vi "Analyze Condition C.vi"(6 "Conditions":T8, 8 "error in":errorcluster, 10 "PLC Data In":T1 {"PLC Data - LDO"."Timing"."Absolute Time" format="%<%H:%M:%S%3u>t"; "PLC Data - LDO"."Timing"."Display Time" format="%#.20f"; "PLC Data - LDO"."Timing"."Test Time Ref" format="%#.20f"; "PLC Data - LDO"."Timing"."Precondition Time Ref" format="%#.20f"; "PLC Data - LDO"."Timing"."First Call Time Ref" format="%#.20f"; "PLC Data - FVIR"."Timing"."Absolute Time" format="%<%H:%M:%S%3u>t"; "PLC Data - FVIR"."Timing"."Display Time" format="%#.20f"; "PLC Data - FVIR"."Timing"."Test Time Ref" format="%#.20f"; "PLC Data - FVIR"."Timing"."Precondition Time Ref" format="%#.20f"; "PLC Data - FVIR"."Timing"."First Call Time Ref" format="%#.20f"}, 11 "Condition Array":dbl[][](array[numeric])) -> (0 "error out":errorcluster, 2 "PLC Data Out":T1 {"PLC Data - LDO"."Timing"."Absolute Time" format="%<%H:%M:%S%3u>t"; "PLC Data - LDO"."Timing"."Display Time" format="%#.20f"; "PLC Data - LDO"."Timing"."Test Time Ref" format="%#.20f"; "PLC Data - LDO"."Timing"."Precondition Time Ref" format="%#.20f"; "PLC Data - LDO"."Timing"."First Call Time Ref" format="%#.20f"; "PLC Data - FVIR"."Timing"."Absolute Time" format="%<%H:%M:%S%3u>t"; "PLC Data - FVIR"."Timing"."Display Time" format="%#.20f"; "PLC Data - FVIR"."Timing"."Test Time Ref" format="%#.20f"; "PLC Data - FVIR"."Timing"."Precondition Time Ref" format="%#.20f"; "PLC Data - FVIR"."Timing"."First Call Time Ref" format="%#.20f"})   [LabVIEW 2020]
uses:
  Terminate Condition ENUM.ctl
  Modbus/Modbus PLC Data All.ctl
  Modbus/Modbus FVIR Control.ctl
  Modbus/Modbus Timing.ctl
  <vilib>/Utility/miscctls.llb/LVDateTimeRec.ctl
  Modbus/Modbus LDO Control.ctl
  WritingDataFile/Data to Save.ctl
  Terminate Conditions Cluster.ctl
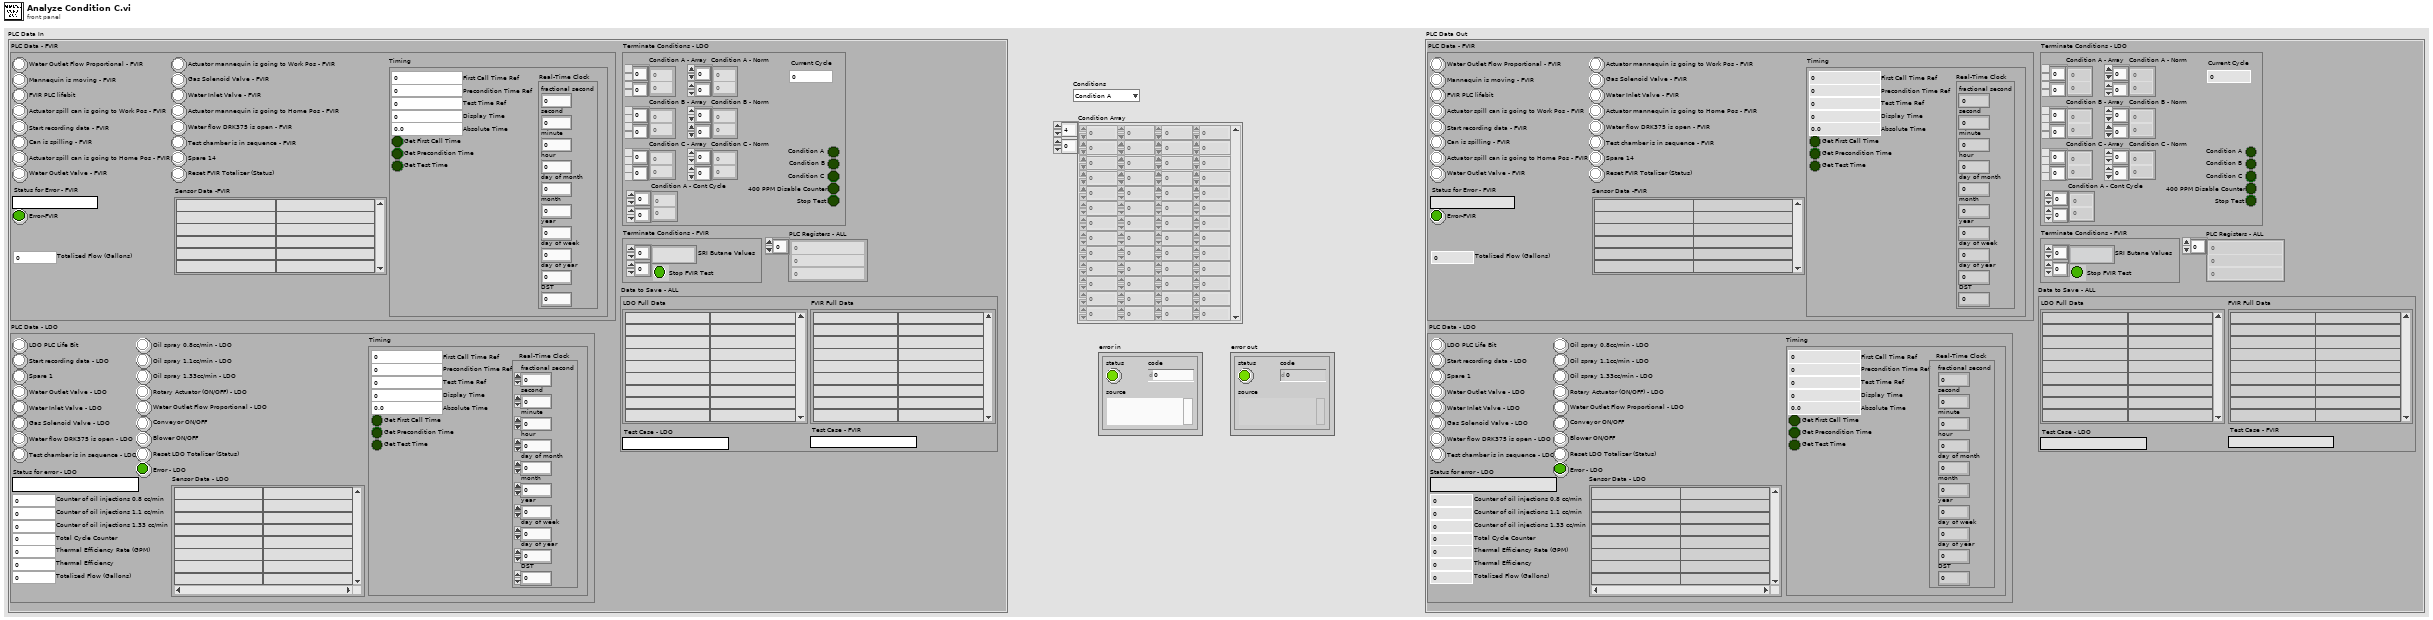
[diagram p1: front panel]
types:
  T1 = typedef "Modbus PLC Data All.ctl" = cluster{"PLC Data - FVIR":T2, "PLC Data - LDO":T5, "PLC Registers - ALL":i16[], "Data to Save - ALL":T6, "Terminate Conditions - LDO":T7, "Terminate Conditions - FVIR":cluster{"SRI Butane Values":string[][], "Stop FVIR Test":bool}}
  T2 = typedef "Modbus FVIR Control.ctl" = cluster{"Reset FVIR Totalizer (Status)":bool, "Spare 14":bool, "Actuator mannequin is going to Work Pos - FVIR":bool, "Actuator mannequin is going to Home Pos - FVIR":bool, "Test chamber is in sequence - FVIR ":bool, "Water flow DRK375 is open - FVIR":bool, "Gas Solenoid Valve - FVIR":bool, "Water Inlet Valve - FVIR":bool, "Water Outlet Flow Proportional - FVIR":bool, "Start recording data - FVIR":bool, "Actuator spill can is going to Work Pos - FVIR":bool, "Actuator spill can is going to Home Pos - FVIR":bool, "Water Outlet Valve - FVIR":bool, "Can is spilling - FVIR":bool, "Mannequin is moving - FVIR":bool, "FVIR PLC lifebit":bool, "Status for Error - FVIR":string, "Error-FVIR":bool, "Sensor Data -FVIR":string[][], "Totalized Flow (Gallons)":dbl, "Timing":T3}
  T3 = typedef "Modbus Timing.ctl" = cluster{"First Call Time Ref":dbl, "Precondition Time Ref":dbl, "Test Time Ref":dbl, "Get First Call Time":bool, "Get Precondition Time":bool, "Get Test Time":bool, "Display Time":dbl, "Real-Time Clock":T4, "Absolute Time":dbl}
  T4 = typedef "LVDateTimeRec.ctl" = cluster{"fractional second":dbl, "second":i32, "minute":i32, "hour":i32, "day of month":i32, "month":i32, "year":i32, "day of week":i32, "day of year":i32, "DST":i32}
  T5 = typedef "Modbus LDO Control.ctl" = cluster{"LDO PLC Life Bit":bool, "Start recording data - LDO":bool, "Spare 1":bool, "Water Outlet Valve - LDO":bool, "Water Inlet Valve - LDO":bool, "Gas Solenoid Valve - LDO":bool, "Water flow DRK375 is open - LDO":bool, "Test chamber is in sequence - LDO":bool, "Oil spray 0.8cc/min - LDO":bool, "Oil spray 1.1cc/min - LDO":bool, "Oil spray 1.33cc/min - LDO":bool, "Rotary Actuator (ON/OFF) - LDO":bool, "Water Outlet Flow Proportional - LDO":bool, "Conveyor ON/OFF":bool, "Blower ON/OFF":bool, "Reset LDO Totalizer (Status)":bool, "Status for error - LDO":string, "Error - LDO":bool, "Sensor Data - LDO":string[][], "Thermal Efficiency Rate (GPM)":dbl, "Thermal Efficiency":dbl, "Totalized Flow (Gallons)":dbl, "Counter of oil injections 1.33 cc/min":u16, "Total Cycle Counter":u16, "Counter of oil injections 1.1 cc/min":u16, "Counter of oil injections 0.8 cc/min":u16, "Timing":T3}
  T6 = typedef "Data to Save.ctl" = cluster{"LDO Full Data":string[][], "FVIR Full Data":string[][], "Test Case - FVIR":string, "Test Case - LDO":string}
  T7 = typedef "Terminate Conditions Cluster.ctl" = cluster{"Condition B - Array":dbl[][], "Current Cycle":u16, "Condition C - Array":dbl[][], "Condition A - Array":dbl[][], "400 PPM Disable Counter":bool, "Condition A - Norm":dbl[][], "Condition B - Norm":dbl[][], "Condition C - Norm":dbl[][], "Condition A":bool, "Condition B":bool, "Condition C":bool, "Condition A - Cont Cycle":dbl[][], "Stop Test":bool}
  T8 = typedef "Terminate Condition ENUM.ctl" = enum16{"Condition A", "Condition B", "Condition C"}
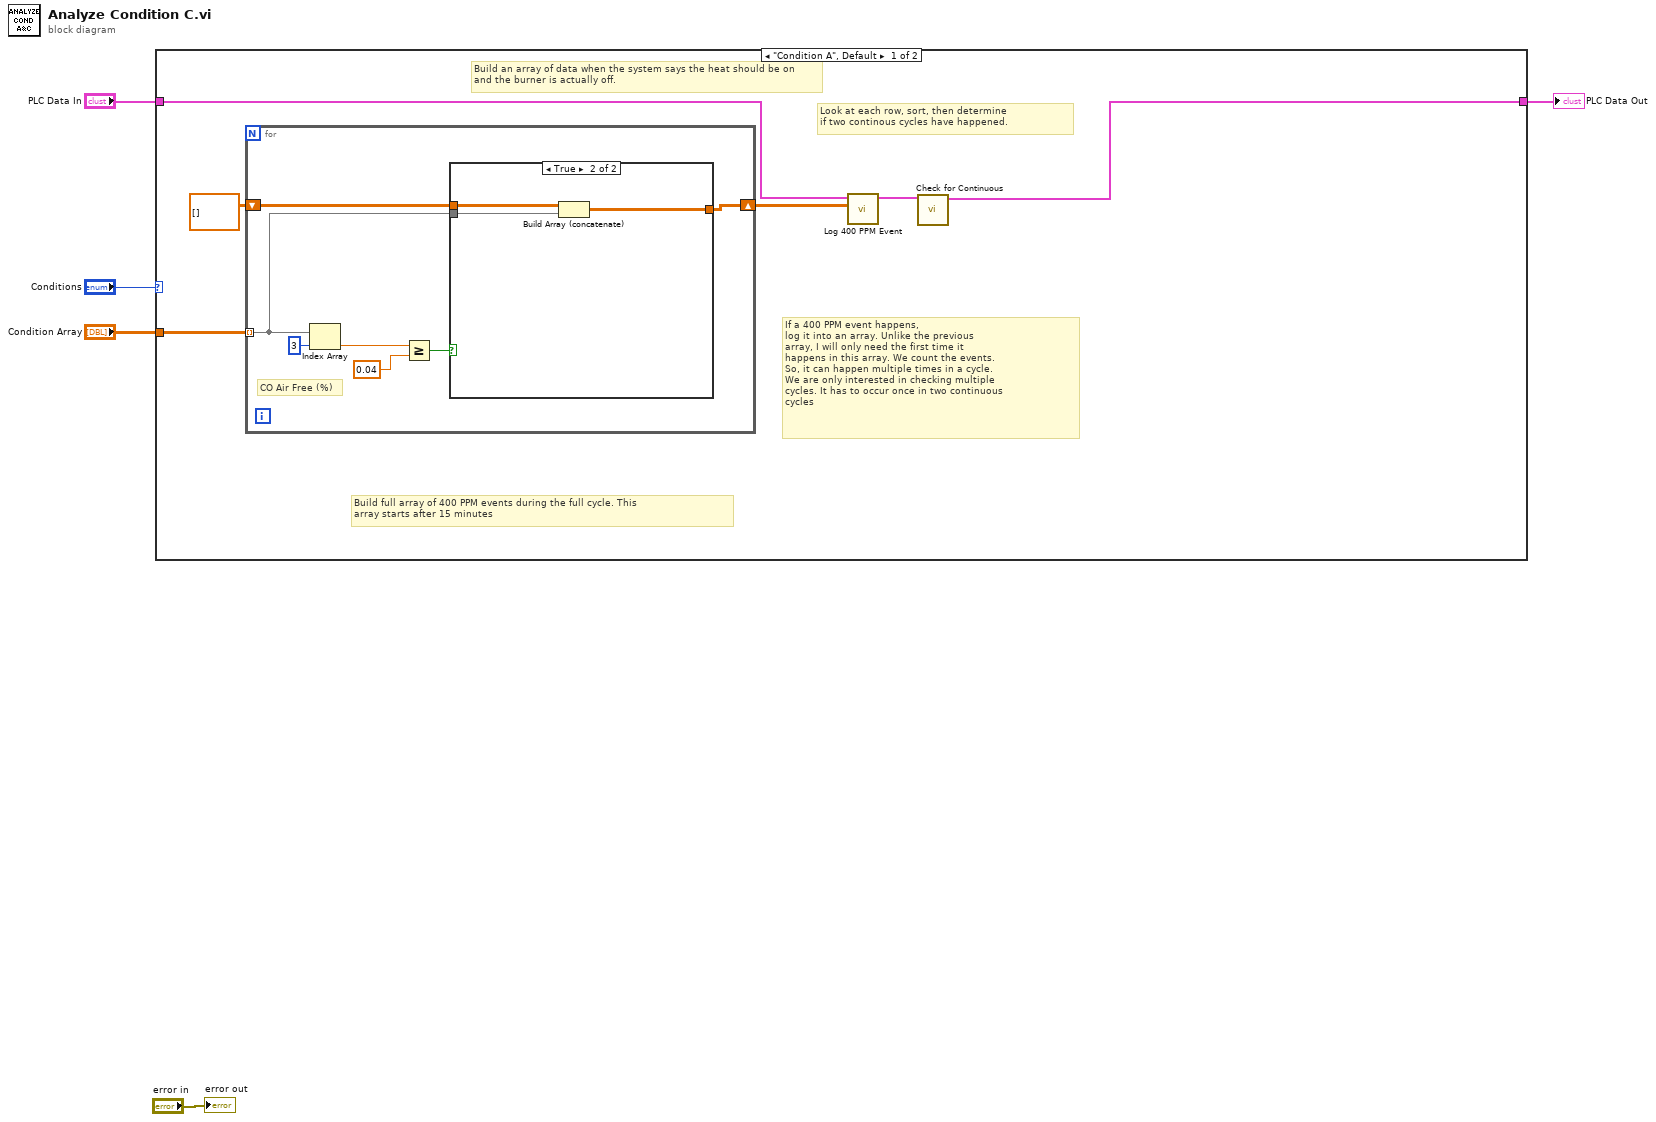
[diagram p0: block diagram]
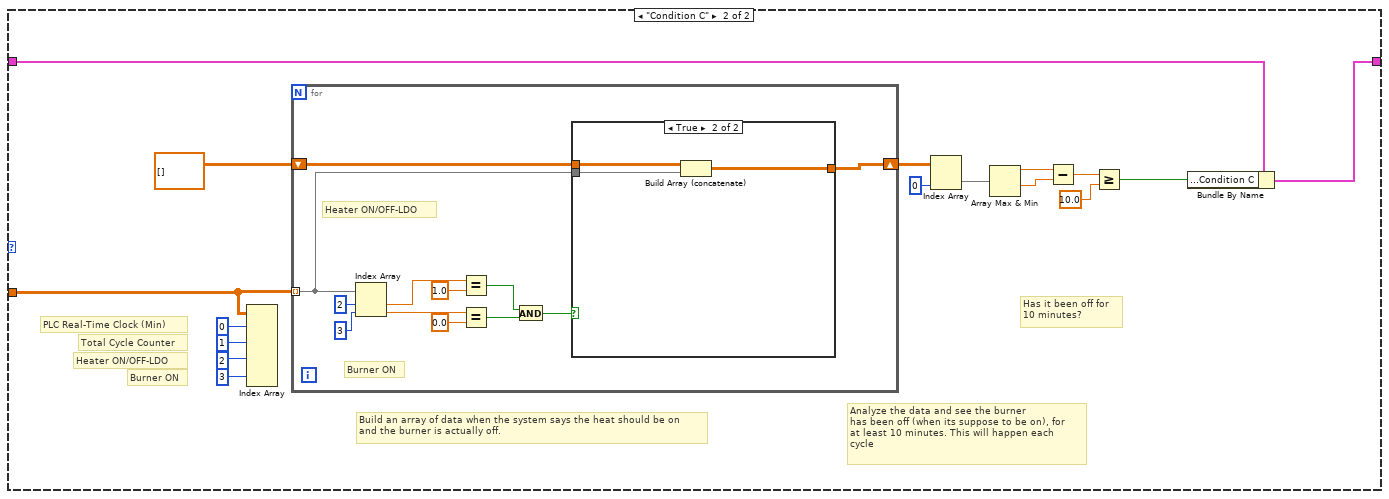
[diagram p3: hidden frame]
diagram:
  n1 = case shown="\"Condition A\", Default" "Conditions" {
    tunnel: "Condition Array" -> [w10 w34]
    tunnel: "PLC Data In" -> [w8 w25]
    tunnel: [w6 w24] -> w1
    frame "Condition A", Default {
      # "Build full array of 400 PPM events during the full cycle. This\narray starts after 15 minutes"
      # "If a 400 PPM event happens,\nlog it into an array. Unlike the previous\narray, I will only need the first time it\nhappens in this array. We count the events.\nSo, it can happen multiple times in a cycle. \nWe are only interested in checking multiple\ncycles. It has to occur once in two continuous\ncycles"
      # "Look at each row, sort, then determine\nif two continous cycles have happened."
      # "Build an array of data when the system says the heat should be on\nand the burner is actually off."
      n2 = for {
        tunnel: w10 -> [w13] mode=indexing
        shift-right: [w14] -> w9
        shift-left: dbl[][] [] -> [w15]
        # "CO Air Free (%)"
        n3 = Index Array(array=w13, index=3) -> (element=w17:dbl)
        n4 = Greater Or Equal?(x=w17, y=0.04) -> (x >= y?=w12:bool)
        n5 = case shown="True" w12 {
          tunnel: w15 -> [w19 w22]
          tunnel: [w19 w21] -> w14
          tunnel: w13 -> [_ w20]
          frame False {
          }
          frame True {
            n6 = Build Array (concatenate)(w22, w20) -> (w21:dbl[][])
          }
        }
      }
      n7 = call "Log 400 PPM Event.vi"("Array"=w9, "PLC Data In in"=w8) -> ("PLC Data In out"=w7:T1)  [unwired: 9 in]
      n8 = call "Check for Continuous.vi"("PLC Data In in"=w7) -> ("PLC Data In out"=w6:T1)  [unwired: 10 in]
    }
    frame "Condition C" {
      # "Analyze the data and see the burner \nhas been off (when its suppose to be on), for\nat least 10 minutes. This will happen each\ncycle"
      # "Build an array of data when the system says the heat should be on\nand the burner is actually off."
      # "Has it been off for \n10 minutes?"
      # "Total Cycle Counter"
      # "PLC Real-Time Clock (Min)"
      # "Burner ON"
      # "Heater ON/OFF-LDO"
      n9 = Index Array(array=w34, index (row) #1=0 ("disabled index (col)"), index (row) #2=1 ("disabled index (col)"), index (row) #3=2 ("disabled index (col)"), index (row) #4=3 ("index (col)")) -> ()  [unwired: 4 in, 4 out]
      n10 = for {
        tunnel: w34 -> [w39] mode=indexing
        shift-right: [w40] -> w32
        shift-left: dbl[][] [] -> [w41]
        # "Burner ON"
        # "Heater ON/OFF-LDO"
        n11 = Index Array(array=w39, index #1=2 ("index"), index #2=3 ("index")) -> (element #1=w48:dbl, element #2=w45:dbl)
        n12 = Equal?(x=w48, y=1.0) -> (x = y?=w44:bool)
        n13 = Equal?(x=w45, y=0.0) -> (x = y?=w43:bool)
        n14 = And(x=w44, y=w43) -> (x .and. y?=w42:bool)
        n15 = case shown="True" w42 {
          tunnel: w41 -> [w51 w54]
          tunnel: [w51 w53] -> w40
          tunnel: w39 -> [_ w52]
          frame False {
          }
          frame True {
            n16 = Build Array (concatenate)(w54, w52) -> (w53:dbl[][])
          }
        }
      }
      n17 = Index Array(array=w32, index (col)=0 ("disabled index (col)")) -> (element=w30:dbl[])  [unwired: 1 in]
      n18 = Array Max & Min(array=w30) -> (max value=w29:dbl, min value=w28:dbl)  [unwired: 2 out]
      n19 = Subtract(x=w29, y=w28) -> (x-y=w27:dbl)
      n20 = Greater Or Equal?(x=w27, y=10.0) -> (x >= y?=w23:bool)
      n21 = Bundle By Name(cluster=w25, "Terminate Conditions - LDO.Condition C"=w23) -> (w24:T1)
    }
  }
  "PLC Data Out" <- w1
  "error out" <- "error in"
